vi "XNET Write (State LIN Schedule Change).vi"(0 "session in":refnum<k21>, 5 "data":refnum<k21>, 11 "error in (no error)":errorcluster) -> (4 "session out":refnum<k21>, 15 "error out":errorcluster)   [LabVIEW 2018]
doc: "Write request for a LIN schedule change.\nThe data can be an XNET LIN Schedule I/O name, or a string that consists of a decimal index to the LIN:Schedules property."
uses:
  nixlvapi.dll
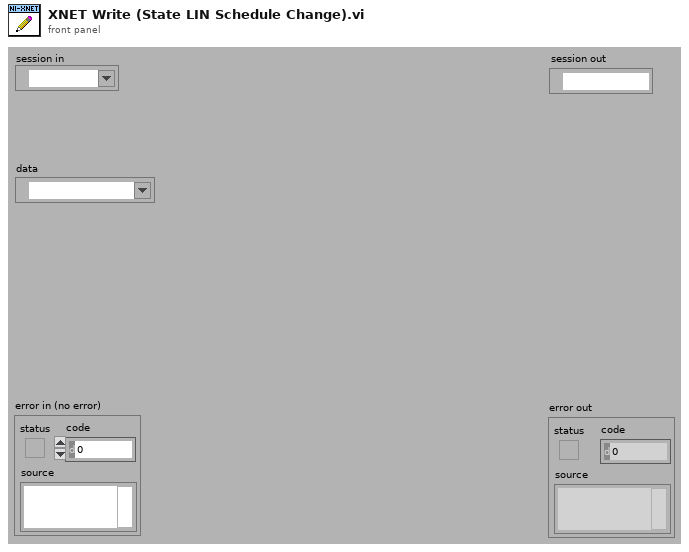
[diagram p1: front panel]
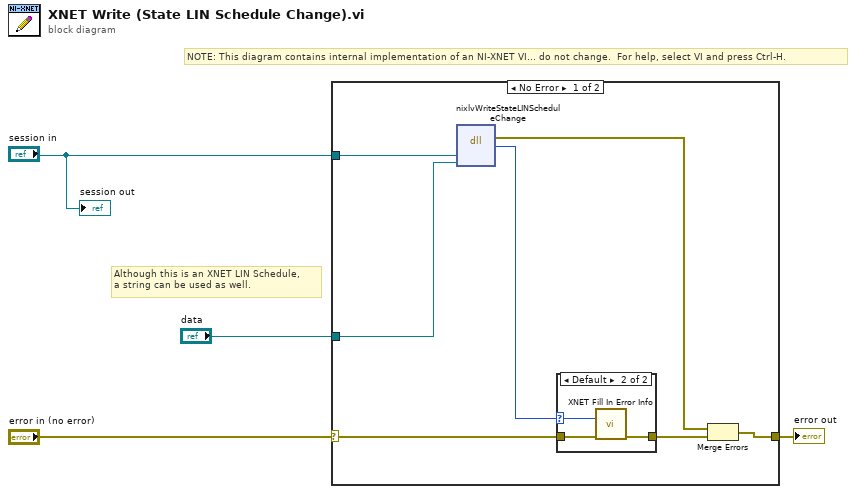
[diagram p0: block diagram]
diagram:
  # "Although this is an XNET LIN Schedule,\na string can be used as well."
  # "NOTE: This diagram contains internal implementation of an NI-XNET VI... do not change.  For help, select VI and press Ctrl-H."
  n1 = case shown="No Error" "error in (no error)" {
    selector: "error in (no error)" -> [w10 w16]
    tunnel: "session in" -> [w11 _]
    tunnel: [w6 w16] -> w4
    tunnel: "data" -> [w7 _]
    frame No Error {
      n2 = dll-call lib="nixlvapi.*" fn="nixlvWriteStateLINScheduleChange"("SessionRef"=w11, "Data"=w7) -> (error out=w5:errorcluster, "return type"=w8:i32)  [unwired: 3 in, 3 out]
      n3 = case shown="Default" w8 {
        selector: w8 -> [_ w13]
        tunnel: w10 -> [w12 w14]
        tunnel: [w12 w15] -> w9
        frame 0 {
        }
        frame Default {
          n4 = call "XNET Fill In Error Info.vi"("status code"=w13, "error in"=w14) -> ("error out"=w15:errorcluster)  [unwired: 13 out]
        }
      }
      n5 = Merge Errors(w5, w9) -> (w6:errorcluster)
    }
    frame Error {
    }
  }
  "error out" <- w4
  "session out" <- "session in"
